vi "AlliGator Find Cursor Connecting Line Intersection(s) with Universal Circle.vi"(8 "Error In":errorcluster, 11 "XY Graph Refnum":refnum<vi>) -> (0 "Error Out":errorcluster, 2 "Intersection 2":cluster{"x":dbl, "y":dbl}, 3 "Intersection 1":cluster{"x":dbl, "y":dbl})   [LabVIEW 2021, in "AlliGator Phasor Graph.lvlib"]
doc: "Computes intersections of a segment connecting the first two cursors of the Phasor Graph with the universal circle."
uses:
  AlliGator Phasor Graph.lvlib
  Math/Math.lvlib
panel:
  # "see the AlliGator License on the block diagram (Ctrl+E or Window:Show Block Diagram)"
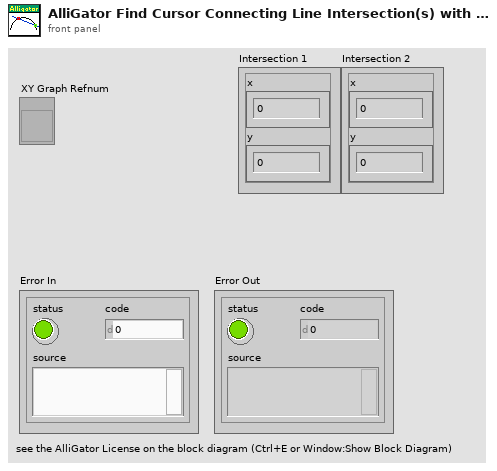
[diagram p1: front panel]
types:
  T1 = typedef "LVCursorListTypeDef.ctl" = cluster{"Name":string, "Color":u32, "Style":u8, "Point Style":u8, "Name Visible":bool, "Allow Drag":bool, "Cursor Mode":u32, "Plot":i32, "Index":i32, "Position":cluster{"X":dbl, "Y":dbl}, "X Scale":u32, "Y Scale":u32, "Watch Plots":i32[], "Watch All Plots":bool, "Plot Area":i32, "Label Offset":cluster{"X":dbl, "Y":dbl}}[]
  T2 = cluster{"Name":string, "Color":u32, "Style":u8, "Point Style":u8, "Name Visible":bool, "Allow Drag":bool, "Cursor Mode":u32, "Plot":i32, "Index":i32, "Position":cluster{"X":dbl, "Y":dbl}, "X Scale":u32, "Y Scale":u32, "Watch Plots":i32[], "Watch All Plots":bool, "Plot Area":i32, "Label Offset":cluster{"X":dbl, "Y":dbl}}
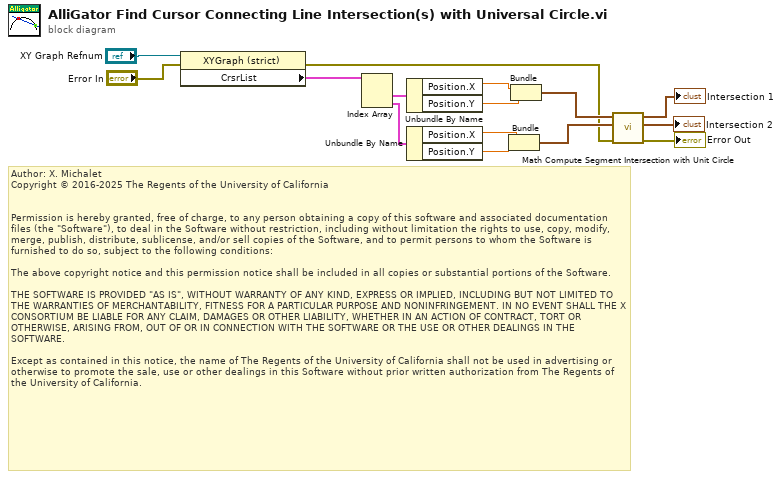
[diagram p0: block diagram]
diagram:
  # "Author: X. Michalet\nCopyright © 2016-2025 The Regents of the University of California\n \n\nPermission is hereby granted, free of charge, to any person obtaining a copy of this software and associated documentation files (the \"Software\"), to deal in the Software without restriction, including without limitation the rights to use, copy, modify, merge, publish, distribute, sublicense, and/or sell copies of the Software, and to permit persons to whom the Software is furnished to do so, subject to the following conditions:\n\nThe above copyright notice and this permission notice shall be included in all copies or substantial portions of the Software.\n\nTHE SOFTWARE IS PROVIDED \"AS IS\", WITHOUT WARRANTY OF ANY KIND, EXPRESS OR IMPLIED, INCLUDING BUT NOT LIMITED TO THE WARRANTIES OF MERCHANTABILITY, FITNESS FOR A PARTICULAR PURPOSE AND NONINFRINGEMENT. IN NO EVENT SHALL THE X CONSORTIUM BE LIABLE FOR ANY CLAIM, DAMAGES OR OTHER LIABILITY, WHETHER IN AN ACTION OF CONTRACT, TORT OR OTHERWISE, ARISING FROM, OUT OF OR IN CONNECTION WITH THE SOFTWARE OR THE USE OR OTHER DEALINGS IN THE SOFTWARE.\n\nExcept as contained in this notice, the name of The Regents of the University of California shall not be used in advertising or otherwise to promote the sale, use or other dealings in this Software without prior written authorization from The Regents of the University of California."
  n1 = property class="XYGraph (strict)"(reference="XY Graph Refnum", error in="Error In") -> (error out=w2:errorcluster, "CrsrList"=w11:T1)  [unwired: 1 out]
  n2 = Index Array(array=w11) -> (element #1=w13:T2, element #2=w12:T2)  [unwired: 2 in]
  n3 = Unbundle By Name(w13) -> ("Position.X"=w7:dbl, "Position.Y"=w6:dbl)
  n4 = Unbundle By Name(w12) -> ("Position.X"=w4:dbl, "Position.Y"=w3:dbl)
  n5 = Bundle("X"=w4, "Y"=w3) -> (w5:cluster{"X":dbl, "Y":dbl})  [unwired: 1 in]
  n6 = Bundle("X"=w7, "Y"=w6) -> (w8:cluster{"X":dbl, "Y":dbl})  [unwired: 1 in]
  n7 = call "Math Compute Segment Intersection with Unit Circle.vi"("Error In"=w2, "Point 2"=w5, "Point 1"=w8) -> ("Error Out"=→"Error Out":errorcluster, "Intersection 2"=→"Intersection 2":cluster{"x1m":dbl, "y1m":dbl}, "Intersection 1"=→"Intersection 1":cluster{"x1p":dbl, "y1p":dbl})  [unwired: 6 in]
